vi "LabVIEW for IBM4 Waveform.vi"() -> ()   [LabVIEW 2021]
uses:
  <vilib>/Instr/_visa.llb/VISA Flush IO Buffer Mask.ctl
  <vilib>/Instr/_visa.llb/VISA Configure Serial Port (Instr).vi
panel:
  out "XY Graph":cluster{i32[], i32[]}(graph)
  out "error out":errorcluster
  in  "write buffer":string
  # "Remember to change your com port to match the port used by your IBM4"
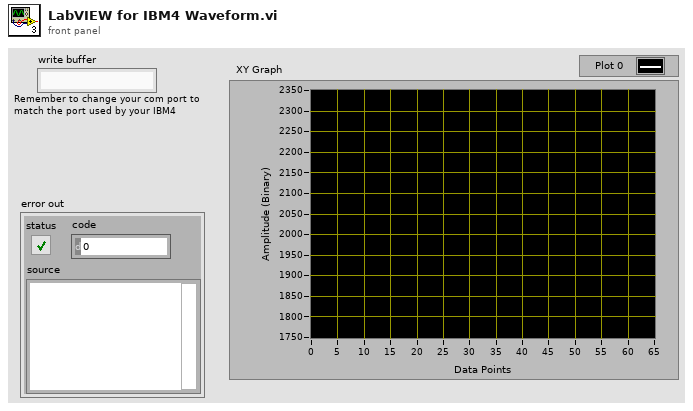
[diagram p1: front panel]
types:
  T1 = typedef "VISA Flush IO Buffer Mask.ctl" = u16
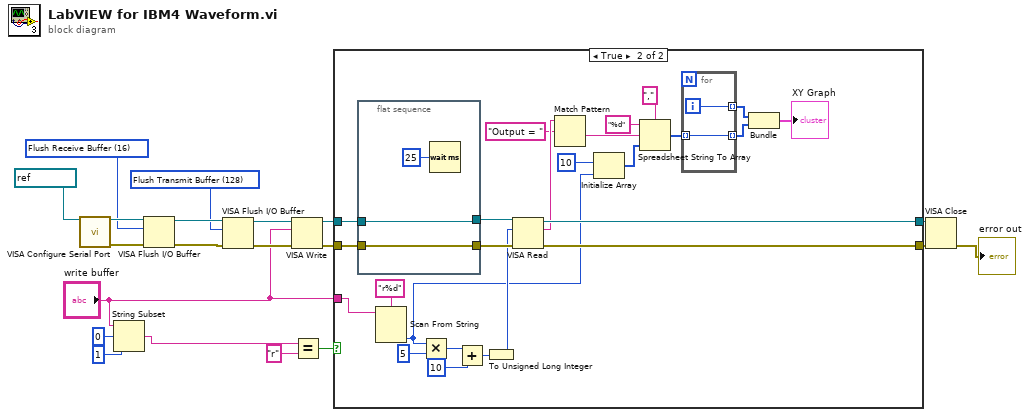
[diagram p0: block diagram]
diagram:
  w14 = T1 128 items=["Flush Receive Buffer"=16, "Write Transmit Buffer to Device"=32, "Flush Receive Buffer (No I/O)"=64, "Flush Transmit Buffer"=128] ("Mask")
  w17 = T1 16 items=["Flush Receive Buffer"=16, "Write Transmit Buffer to Device"=32, "Flush Receive Buffer (No I/O)"=64, "Flush Transmit Buffer"=128] ("Mask")
  n1 = call-poly "VISA Configure Serial Port"("VISA resource name"=refnum<visa-resource-name> "COM9") -> ("VISA resource name out"=w19:refnum<visa-resource-name>, "error out"=w18:errorcluster)  [unwired: 13 in]
  n2 = String Subset(string="write buffer", offset (0)=0, length (rest)=1 ("length (rest)")) -> (substring=w3:string)
  n3 = VISA Flush I/O Buffer(VISA resource name=w19, mask (16)=w17, error in (no error)=w18) -> (VISA resource name out=w16:refnum<visa-resource-name>, error out=w15:errorcluster)
  n4 = VISA Flush I/O Buffer(VISA resource name=w16, mask (16)=w14, error in (no error)=w15) -> (VISA resource name out=w13:refnum<visa-resource-name>, error out=w12:errorcluster)
  n5 = VISA Write(VISA resource name=w13, write buffer="write buffer", error in (no error)=w12) -> (VISA resource name out=w8:refnum<visa-resource-name>, error out=w7:errorcluster)  [unwired: 1 out]
  n6 = Equal?(x=w3, y="r") -> (x = y?=w4:bool)
  n7 = case shown="True" w4 {
    tunnel: [w21 w47] -> w11
    tunnel: [w22 w46] -> w10
    tunnel: w8 -> [w22 w45]
    tunnel: w7 -> [w21 w43]
    tunnel: "write buffer" -> [_ w41]
    frame False {
    }
    frame True {
      n8 = flat-sequence {
        tunnel: [w52] -> w44
        tunnel: w45 -> [w52]
        tunnel: [w51] -> w42
        tunnel: w43 -> [w51]
        frame #0 {
          n9 = Wait (ms)(milliseconds to wait=u32 25) -> ()  [unwired: 1 out]
        }
      }
      n10 = Scan From String(format string="r%d", input string=w41) -> (output 1=w28:i32)  [unwired: 3 in, 3 out]
      n11 = Multiply(x=w28, y=5) -> (x*y=w38:i32)
      n12 = Add(x=w38, y=10) -> (x+y=w36:i32)
      n13 = To Unsigned Long Integer(number=w36) -> (unsigned 32bit integer=w35:u32)
      n14 = VISA Read(VISA resource name=w44, byte count=w35, error in (no error)=w42) -> (VISA resource name out=w46:refnum<visa-resource-name>, read buffer=w34:string, error out=w47:errorcluster)  [unwired: 1 out]
      n15 = Match Pattern(string=w34, regular expression="Output = ") -> (after substring=w32:string)  [unwired: 1 in, 3 out]
      n16 = Initialize Array(10 ("y"), w28) -> (w27:i32[])
      n17 = Spreadsheet String To Array(delimiter (Tab)=",", format string="%d", spreadsheet string=w32, array type (2D Dbl)=w27) -> (array=w26:i32[])
      n18 = for {
        tunnel: w26 -> [w49] mode=indexing
        tunnel: [w49] -> w23 mode=indexing
        tunnel: [w48] -> w25 mode=indexing
        i -> [w48]
      }
      n19 = Bundle(w25, w23) -> (→"XY Graph":cluster{i32[], i32[]})  [unwired: 1 in]
    }
  }
  n20 = VISA Close(VISA resource name=w10, error in (no error)=w11) -> (error out=→"error out":errorcluster)
